vi "(SubVI) Write and Read Waveform.vi"(4 "ADC Rate (Read)(ms)":dbl=1.0 min=0.033333 max=5.0 format="%.4f", 5 "Data Array In to write":dbl[](array[numeric]) format="%.2f", 6 "Number of Positions to Read":u32=2 min=2 max=10000, 9 "DAC Rate (Write) (ms)":dbl=1.0 min=0.0333333 max=5.0 format="%.4f", 10 "handle":i32, 11 "Axis":u32) -> (2 "Data Array Out to read":dbl[](array[numeric]) format="%.2f")   [LabVIEW 2014]
uses:
  MCL-dll-Labview 32-bit/Madlib.dll
panel:
  out "Return Code":i32
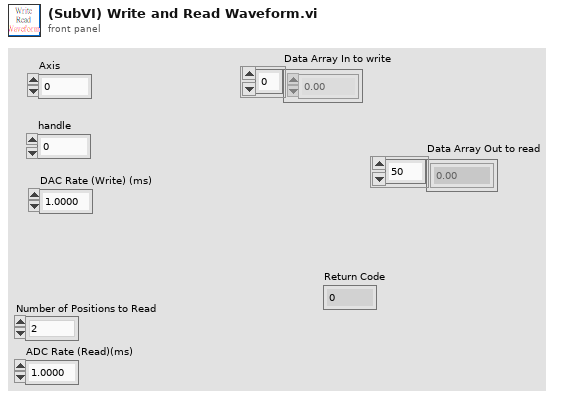
[diagram p1: front panel]
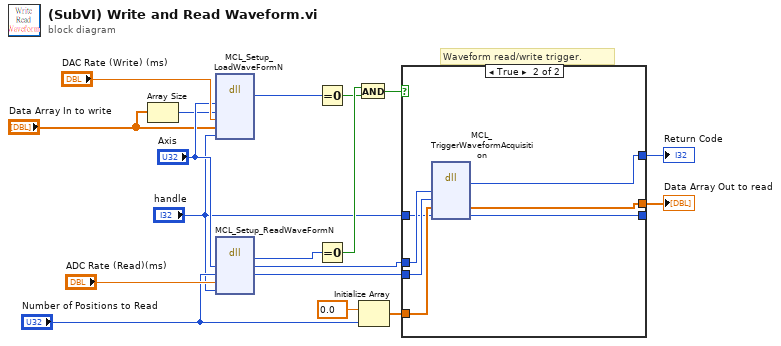
[diagram p0: block diagram]
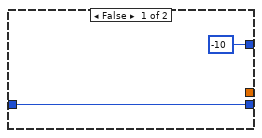
[diagram p2: hidden frame]
diagram:
  # "Waveform read/write trigger."
  n1 = Array Size(array="Data Array In to write") -> (size(s)=w1:i32)
  n2 = dll-call lib="C:/Users/OT-hwlab/Desktop/YCC's OT/Main-Stage-Based/SubVI-Stage-Based/MCL-dll-Labview 32-bit/Madlib.dll" fn="MCL_Setup_LoadWaveFormN" label="Setup WF Load"("axis"="Axis", "DataPoints"=w1, "milliseconds"="DAC Rate (Write) (ms)", "waveform"="Data Array In to write", "handle"="handle") -> ("return type"=w12:i32)  [unwired: 8 in, 2 out]
  n3 = dll-call lib="C:/Users/OT-hwlab/Desktop/YCC's OT/Main-Stage-Based/SubVI-Stage-Based/MCL-dll-Labview 32-bit/Madlib.dll" fn="MCL_Setup_ReadWaveFormN" label="Setup WF Read"("axis"="Axis", "DataPoints"="Number of Positions to Read", "milliseconds"="ADC Rate (Read)(ms)", "handle"="handle") -> ("return type"=w13:i32, "axis"=w16:u32, "DataPoints"=w15:u32)  [unwired: 5 in, 2 out]
  n4 = Equal To 0?(x=w12) -> (x = 0?=w17:bool)
  n5 = Equal To 0?(x=w13) -> (x = 0?=w18:bool)
  n6 = And(x=w18, y=w17) -> (x .and. y?=w14:bool)
  n7 = Initialize Array(0.0, "Number of Positions to Read") -> (w8:dbl[])
  n8 = case shown="True" w14 {
    tunnel: [_ w27] -> w4
    tunnel: w16 -> [_ w26]
    tunnel: w15 -> [_ w25]
    tunnel: w8 -> [_ w24]
    tunnel: "handle" -> [w20 w23]
    tunnel: [w20 w22] -> _
    tunnel: [-10 w21] -> w5
    frame False {
    }
    frame True {
      n9 = dll-call lib="C:/Users/OT-hwlab/Desktop/YCC's OT/Main-Stage-Based/SubVI-Stage-Based/MCL-dll-Labview 32-bit/Madlib.dll" fn="MCL_TriggerWaveformAcquisition"("axis"=w26, "DataPoints"=w25, "waveform"=w24, "handle"=w23) -> ("return type"=w21:i32, "waveform"=w27:dbl[], "handle"=w22:i32)  [unwired: 5 in, 2 out]
    }
  }
  "Data Array Out to read" <- w4
  "Return Code" <- w5
